vi "Reload Sub Panel.vi"(8 "error in (no error)":errorcluster, 10 "sub panel":refnum<vi>, 11 "[V] Waveform in":refnum<class "[V] Waveform.lvclass">) -> (0 "error out":errorcluster, 3 "[V] Waveform out":refnum<class "[V] Waveform.lvclass">)   [LabVIEW 2023, in "[V] Waveform.lvlib" / "[V] Waveform.lvclass"]
uses:
  [V] Waveform.lvclass
  [V] Waveform.lvclass/[V] Waveform.ctl
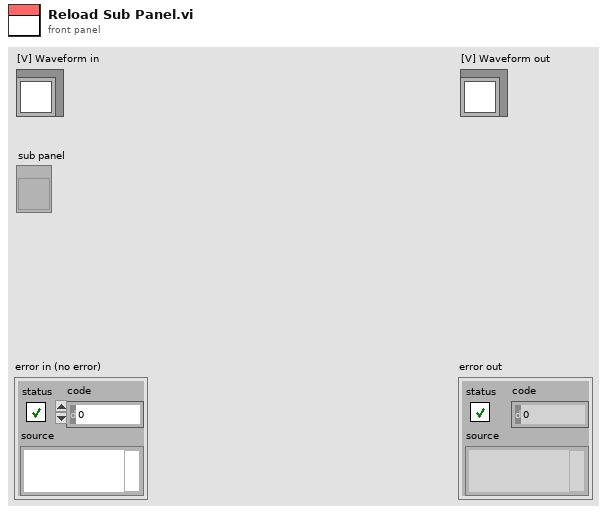
[diagram p1: front panel]
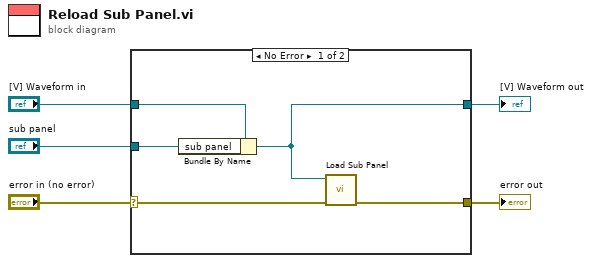
[diagram p0: block diagram]
diagram:
  n1 = case shown="No Error" "error in (no error)" {
    selector: "error in (no error)" -> [w8 w12]
    tunnel: [w6 w12] -> w4
    tunnel: [w7 w11] -> w2
    tunnel: "[V] Waveform in" -> [w10 w11]
    tunnel: "sub panel" -> [w9 _]
    frame No Error {
      n2 = Bundle By Name(cluster=w10, "sub panel"=w9) -> (w7:refnum<class "[V] Waveform.lvclass">)
      n3 = call "Load Sub Panel.vi"("error in (no error)"=w8, "[V] Waveform in"=w7) -> ("error out"=w6:errorcluster)  [unwired: 8 in, 1 out]
    }
    frame Error {
    }
  }
  "error out" <- w4
  "[V] Waveform out" <- w2
